vi "ConfigureTrig.vi"(8 "error in (no error)":errorcluster, 11 "reference in":refnum<class "sim_MmW.lvclass">) -> (0 "error out":errorcluster, 3 "reference out":refnum<class "sim_MmW.lvclass">)   [LabVIEW 2019, in "sim_MmW.lvclass"]
uses:
  sim_MmW.lvclass
  C:/Barkhausen mmWave radar/Development/modules/mmw_instrument/src_LabVIEW/Host/SubVIs/mmWave instrument_class/mmWave instrument.lvclass
  mmWave instrument_class/mmWave instrument.lvclass
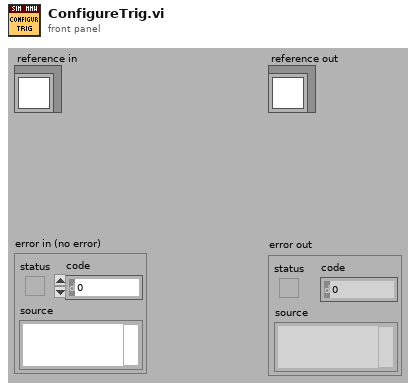
[diagram p1: front panel]
types:
  T1 = typedef "sim_MmW.lvclass/ObjectAttributesRef.ctl" = refnum<data-value>
  T2 = typedef "mmWave instrument.lvclass/ObjectAttributes.ctl" = cluster{"mode":T3, "instr state":T4, "Max Fs":dbl, "Equalization coeff":cdb[], "LO sync en":bool, "Trig sync en":bool, "LO sources":T5, "LO Export":T6, "Fc.range":cluster{"min":dbl, "max":dbl}, "Sync mode":T7, "equalization en":bool, "sequence":string[]}
  T3 = typedef "mmWave instrument.lvclass/Instrument mode.ctl" = enum16{"RF", "IF", "BB"}
  T4 = typedef "mmWave instrument.lvclass/Instrument state.ctl" = enum16{"Off", "Initialization", "Configuration", "Running", "Calibration"}
  T5 = typedef "mmWave HW Control.lvlib/LO sources.ctl" = cluster{"RX/LO1 src":string, "TX/LO1 src":string, "LO2 src":string}
  T6 = typedef "mmWave HW Control.lvlib/LO export.ctl" = cluster{"TX LO1 export":bool, "TX LO1 export level":dbl, "RX LO1 export":bool, "RX LO1 export level":dbl, "LO2 export":bool, "LO2 export level":dbl}
  T7 = typedef "mmWave instrument.lvclass/Sync mode.ctl" = enum16{"Slave", "Master"}
  T8 = typedef "sim_MmW.lvclass/ObjectAttributes.ctl" = cluster{"RF config":T9, "RX samples":i32, "Downloaded Bursts":map{string, refnum<class "mmWave data.lvclass">}, "TX Fs":dbl, "RX Fs":dbl, "burst sequence":string[], "Burst mode":T10}
  T9 = typedef "mmWave HW Control.lvlib/HW TXRX RF config cluster.ctl" = cluster{"TX.Frequency":dbl, "TX.Gain":dbl, "TX.mmWave adapter":string, "RX.Frequency":dbl, "RX.Gain":dbl, "RX.mmWave adapter":string}
  T10 = typedef "mmWave instrument.lvclass/BurstMode.ctl" = enum16{"burst", "continuous"}
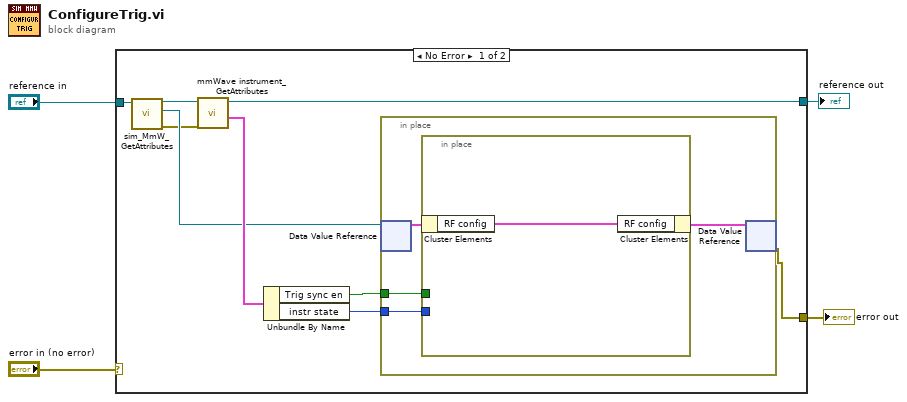
[diagram p0: block diagram]
diagram:
  n1 = case shown="No Error" "error in (no error)" {
    selector: "error in (no error)" -> [_ w20]
    tunnel: [w5 w20] -> w3
    tunnel: [w11 w19] -> w1
    tunnel: "reference in" -> [w12 w19]
    frame No Error {
      n2 = call "sim_MmW_GetAttributes.vi"("reference in"=w12) -> ("error out"=w8:errorcluster, "attributes ref"=w9:T1, "reference out"=w13:refnum<class "sim_MmW.lvclass">)  [unwired: 7 in, 1 out]
      n3 = call "mmWave instrument_GetAttributes.vi"("error in (no error)"=w8, "reference in"=w13) -> ("attributes"=w10:T2, "reference out"=w11:refnum<class "sim_MmW.lvclass">)  [unwired: 6 in, 2 out]
      n4 = Unbundle By Name(w10) -> ("Trig sync en"=w6:bool, "instr state"=w7:T4)
      n5 = in-place {
        in-place-border: w7 -> [w15]
        in-place-border: w6 -> [w14]
        n6 = in-place-dvr #1(w9) -> (w17:T8)  [unwired: 1 out]
        n7 = in-place {
          in-place-border: w15 -> [_]
          in-place-border: w14 -> [_]
          n8 = in-place-cluster #2(w17) -> ("RF config"=w18:T9)
          n9 = in-place-cluster #2("RF config"=w18) -> (w16:T8)
        }
        n10 = in-place-dvr #1(w16) -> (w5:errorcluster)  [unwired: 1 out]
      }
    }
    frame Error {
    }
  }
  "error out" <- w3
  "reference out" <- w1
